vi "global_normalize.vi"(10 "trunc_transmission[r=wl, c=v]":dbl[][](array[numeric])) -> (2 "normalized transmission[r=wl, c=v]":dbl[][](array[numeric]))   [LabVIEW 2019]
uses:
  REFS.vi
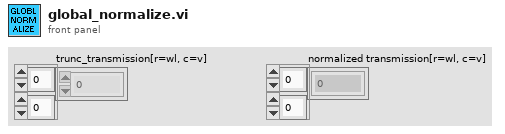
[diagram p1: front panel]
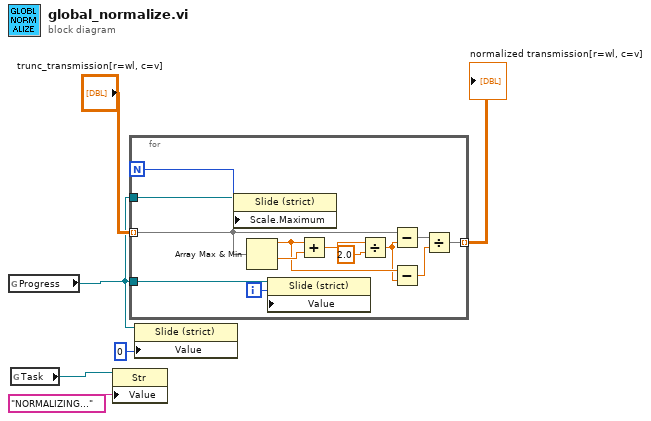
[diagram p0: block diagram]
diagram:
  n1 = global read "REFS.vi" "Progress"() -> (w2:refnum<vi>)
  n2 = global read "REFS.vi" "Task"() -> (w1:refnum<vi>)
  n3 = property class="Str"(reference=w1, "Value"="NORMALIZING...") -> ()  [unwired: 1 in, 2 out]
  n4 = for {
    N -> [w9]
    tunnel: "trunc_transmission[r=wl, c=v]" -> [w15] mode=indexing
    tunnel: [w13] -> w4 mode=indexing
    tunnel: w2 -> [w8]
    tunnel: w2 -> [w7]
    i -> [w10]
    n5 = property on="Property Node" class="Slide (strict)"(reference=w7, "Scale.Maximum"=w9) -> ()  [unwired: 1 in, 2 out]
    n6 = Array Max & Min(array=w15) -> (max value=w16:dbl, min value=w17:dbl)  [unwired: 2 out]
    n7 = property class="Slide (strict)"(reference=w8, "Value"=w10) -> ()  [unwired: 1 in, 2 out]
    n8 = Add(x=w16, y=w17) -> (x+y=w19:dbl)
    n9 = Divide(x=w19, y=2.0) -> (x/y=w12:dbl)
    n10 = Subtract(x=w15, y=w12) -> (x-y=w14:dbl[])
    n11 = Subtract(x=w16, y=w12) -> (x-y=w11:dbl)
    n12 = Divide(x=w14, y=w11) -> (x/y=w13:dbl[])
  }
  "normalized transmission[r=wl, c=v]" <- w4
  n13 = property class="Slide (strict)"(reference=w2, "Value"=0) -> ()  [unwired: 1 in, 2 out]
